vi "mS Timer+.vi"(8 "Error In":errorcluster) -> (0 "Error Out":errorcluster, 3 "MilliSecond Timer Value":dbl format="%_6e")   [LabVIEW 2020]
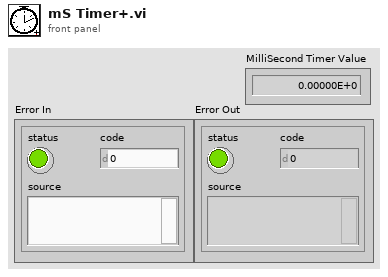
[diagram p1: front panel]
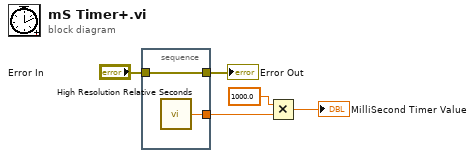
[diagram p0: block diagram]
diagram:
  n1 = stacked-sequence {
    tunnel: [w7] -> w5
    tunnel: "Error In" -> [w7]
    tunnel: [w6] -> w4
    frame #0 {
      n2 = call <vilib>:"High Resolution Relative Seconds.vi"() -> ("relative seconds"=w6:dbl)
    }
  }
  "Error Out" <- w5
  n3 = Multiply(x=1000.0 ("y"), y=w4) -> (x*y=→"MilliSecond Timer Value":dbl)
